vi "BlockSyncStart.vi"(1 "S1":u8, 2 "S2":u8) -> ()   [LabVIEW 2015]
uses:
  ESLSCDLL.dll
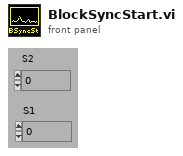
[diagram p1: front panel]
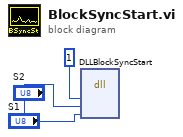
[diagram p0: block diagram]
diagram:
  n1 = dll-call lib="C:/ENTW/PCIE/lv64/board.vis/ESLSCDLL.dll" fn="DLLBlockSyncStart" ("lwlscdll.dll:DLLWriteLongS0")("drv"=u32 1, "S1"="S1", "S2"="S1") -> ()  [unwired: 7 in, 2 out]
